vi "Get BrowerSymbolIndex.vi"(8 "error in (no error)":errorcluster, 11 "BrowerComponent in":refnum<class "BrowerComponent.lvclass">) -> (0 "error out":errorcluster, 2 "SymbolIndex":i32, 3 "BrowerComponent out":refnum<class "BrowerComponent.lvclass">)   [LabVIEW 2015, in "BrowerComponent.lvclass"]
uses:
  BrowerComponent.lvclass
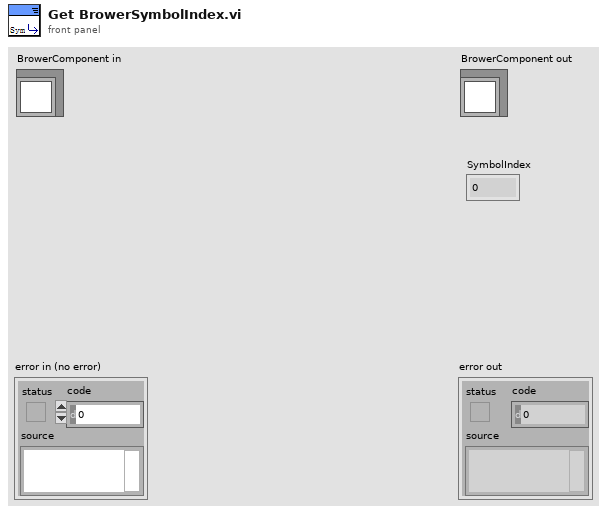
[diagram p1: front panel]
types:
  T1 = typedef "BrowerComponent.lvclass/ObjectAttributes.ctl" = cluster{"ComponentID":string, "SymbolIndex":i32, "ComponentName":string, "PartsOfComponent_dict":variant}
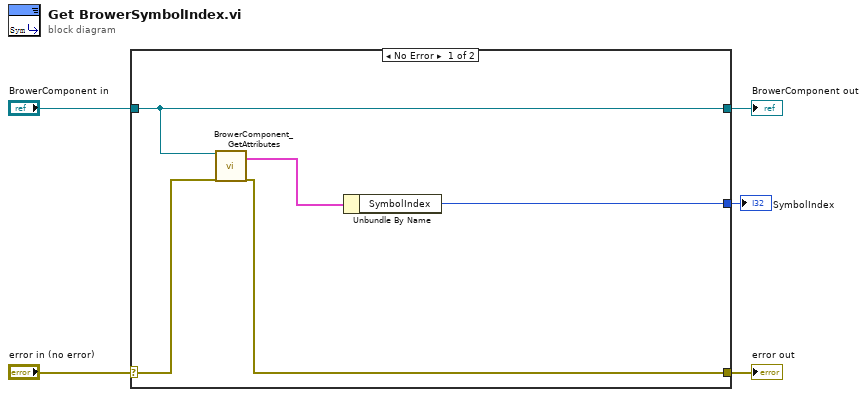
[diagram p0: block diagram]
diagram:
  n1 = case shown="No Error" "error in (no error)" {
    selector: "error in (no error)" -> [w9 w12]
    tunnel: [w6 w12] -> w4
    tunnel: [w10 w11] -> w2
    tunnel: "BrowerComponent in" -> [w10 w11]
    tunnel: [w7 _] -> w1
    frame No Error {
      n2 = call "BrowerComponent_GetAttributes.vi"("reference in"=w10, "error in (no error)"=w9) -> ("Data"=w8:T1, "error out"=w6:errorcluster)  [unwired: 14 in, 2 out]
      n3 = Unbundle By Name(w8) -> ("SymbolIndex"=w7:i32)
    }
    frame Error {
    }
  }
  "error out" <- w4
  "BrowerComponent out" <- w2
  "SymbolIndex" <- w1
